vi "Report Start Build.vi"(6 "Build in":refnum<class "Build.lvclass">, 8 "error in (no error)":errorcluster, 9 "Build Info":T1, 10 "Build Events API in":refnum<class "Build Events API.lvclass">) -> (0 "error out":errorcluster, 2 "Build Events API out":refnum<class "Build Events API.lvclass">)   [LabVIEW 2020, in "Builder Tools.lvlib" / "Builder.lvclass"]
uses:
  Builder.lvclass
  Build Events API/Build Events API.lvclass
  Build Info.ctl
  Build/Build.lvclass
  Builder.lvclass/Builder.ctl
  Builder Tools.lvlib
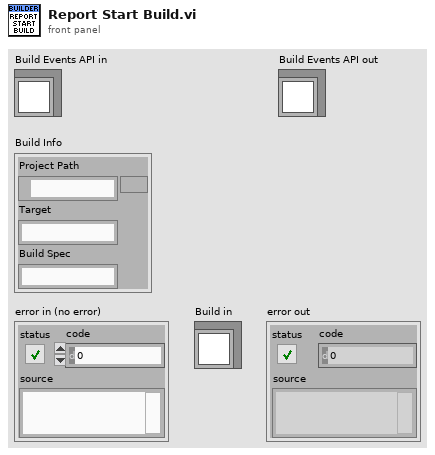
[diagram p1: front panel]
types:
  T1 = typedef "Builder Tools.lvlib/Build Info.ctl" = cluster{"Project Path":path, "Target":string, "Build Spec":string}
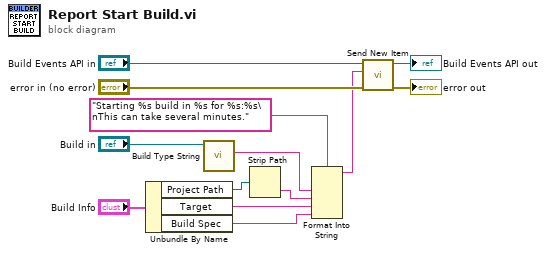
[diagram p0: block diagram]
diagram:
  n1 = Unbundle By Name("Build Info") -> ("Project Path"=w10:path, "Target"=w6:string, "Build Spec"=w5:string)
  n2 = call-dynamic "Build Type String.vi"("Build in"="Build in") -> ("Build Type"=w8:string)  [unwired: 10 in]
  n3 = Strip Path(path=w10) -> (name=w7:string)  [unwired: 1 out]
  n4 = Format Into String(format string="Starting %s build in %s for %s:%s\nThis can take several minutes.", w8, w7, w6, w5) -> (resulting string=w3:string)  [unwired: 2 in, 1 out]
  n5 = call "Send New Item.vi"("error in (no error)"="error in (no error)", "Message"=w3, "Build Events API in"="Build Events API in") -> ("error out"=→"error out":errorcluster, "Build Events API out"=→"Build Events API out":refnum<class "Build Events API.lvclass">)  [unwired: 7 in]
